vi "Write Status String.vi"(8 "error in (no error)":errorcluster, 10 "Camera Status":T1, 11 "RxTxCamera in":refnum<class "RxTxCamera.lvclass">) -> (0 "error out":errorcluster, 3 "RxTxCamera out":refnum<class "RxTxCamera.lvclass">)   [LabVIEW 2018, in "RxTxCamera.lvclass"]
doc: "Este VI recebe um cluter contendo o status da câmera e constrói a string do status da câmera com a tag STATUS na primeira linha."
uses:
  RxTxCamera.lvclass
  C:/Users/Cliente/Desktop/Software Echarpe/RxTx/RxTx.lvclass
  RxTxCamera.lvclass/RxTxCamera.ctl
  RxTx/RxTx.lvclass/RxTx.ctl
  Construct String Camera Status/Construct String Camera Status.lvclass
  RxTx/RxTx.lvclass
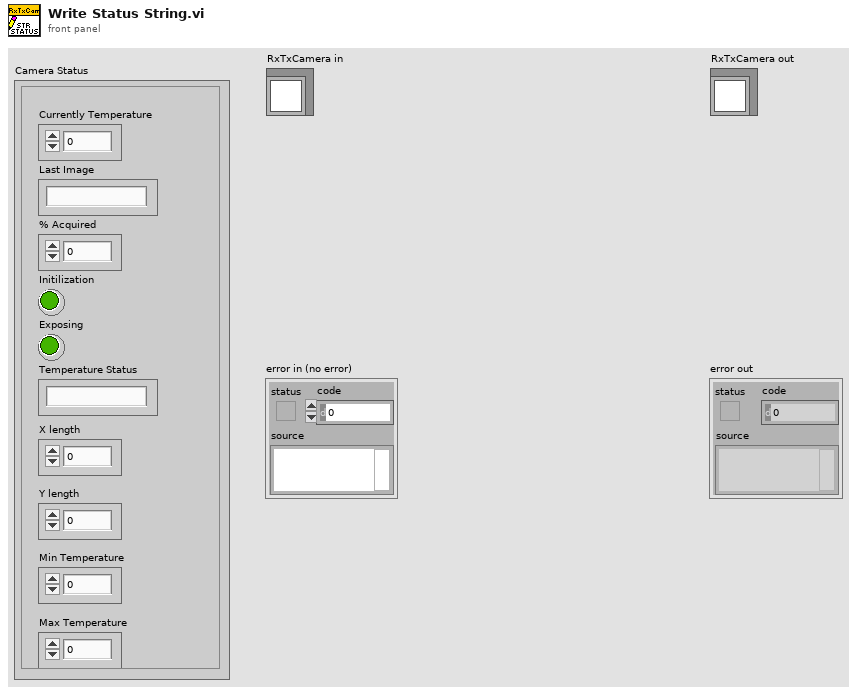
[diagram p1: front panel]
types:
  T1 = cluster{"Currently Temperature":dbl, "Last Image":string, "% Acquired":dbl, "Initilization":bool, "Exposing":bool, "Temperature Status":string, "X length":dbl, "Y length":dbl, "Min Temperature":dbl, "Max Temperature":dbl}
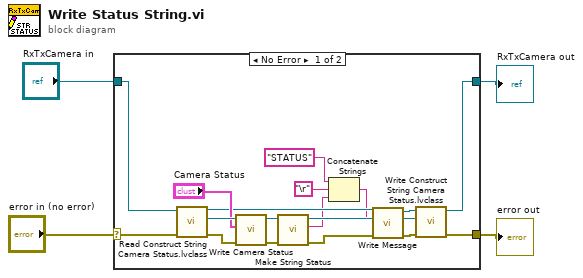
[diagram p0: block diagram]
diagram:
  n1 = case shown="No Error" "error in (no error)" {
    selector: "error in (no error)" -> [w22 w23]
    tunnel: [w19 w23] -> w3
    tunnel: [w20 w24] -> w1
    tunnel: "RxTxCamera in" -> [w21 w24]
    frame No Error {
      n2 = call "Read Construct String Camera Status.lvclass.vi"("error in (no error)"=w22, "RxTxCamera in"=w21) -> ("error out"=w17:errorcluster, "Construct String Camera Status.lvclass"=w16:refnum<class "Construct String Camera Status.lvclass">, "RxTxCamera out"=w9:refnum<class "RxTxCamera.lvclass">)  [unwired: 7 in]
      n3 = call "Write Camera Status.vi"("error in (no error)"=w17, "Camera Status"="Camera Status", "Construct String Camera Status in"=w16) -> ("error out"=w18:errorcluster, "Construct String Camera Status out"=w15:refnum<class "Construct String Camera Status.lvclass">)  [unwired: 7 in]
      n4 = call "Make String Status.vi"("error in (no error)"=w18, "Construct String Camera Status in"=w15) -> ("error out"=w10:errorcluster, "String Camera Status"=w6:string, "Construct String Camera Status out"=w14:refnum<class "Construct String Camera Status.lvclass">)  [unwired: 7 in]
      n5 = Concatenate Strings("STATUS", "\r", w6) -> (w8:string)
      n6 = call "Write Message.vi"("error in (no error)"=w10, "Message"=w8, "RxTx in"=w9) -> ("error out"=w12:errorcluster, "RxTx out"=w11:refnum<class "RxTxCamera.lvclass">)  [unwired: 7 in]
      n7 = call "Write Construct String Camera Status.lvclass.vi"("error in (no error)"=w12, "Construct String Camera Status.lvclass"=w14, "RxTxCamera in"=w11) -> ("error out"=w19:errorcluster, "RxTxCamera out"=w20:refnum<class "RxTxCamera.lvclass">)  [unwired: 7 in]
    }
    frame Error {
    }
  }
  "error out" <- w3
  "RxTxCamera out" <- w1
